vi "Auton Lift Dictation.vi"(1 "Level":dbl, 2 "First Iteration":bool) -> (0 "Lift Sequence Done":bool)   [LabVIEW 2014]
uses:
  Begin/Global Variables.vi
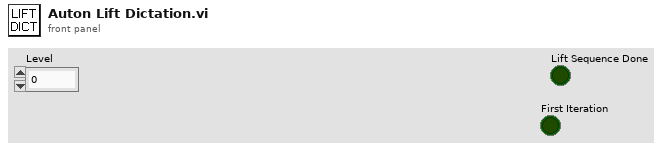
[diagram p1: front panel]
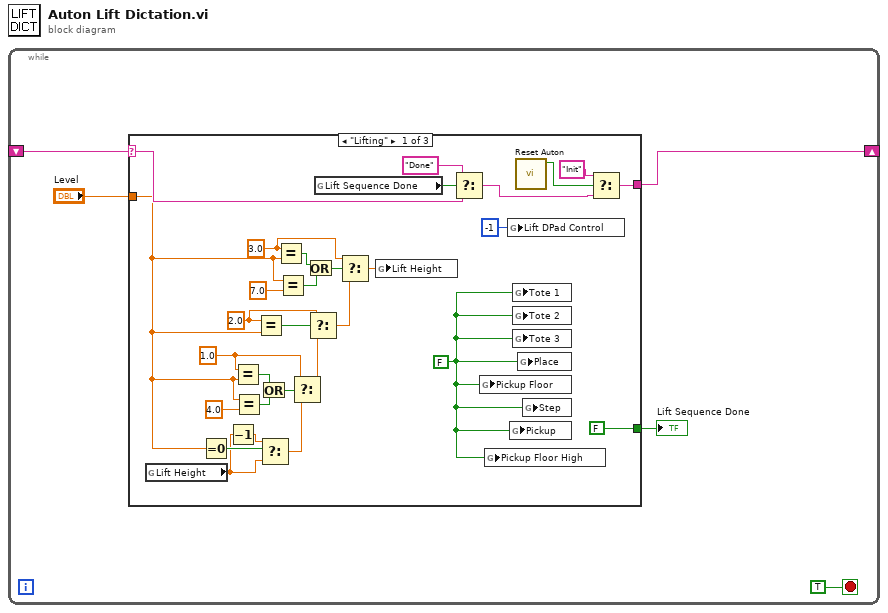
[diagram p0: block diagram]
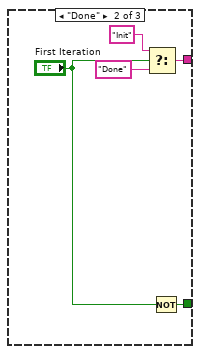
[diagram p2: hidden frame]
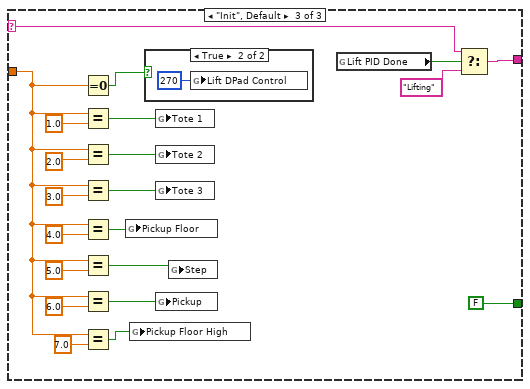
[diagram p3: hidden frame]
diagram:
  n1 = while {
    shift-right: [w1] -> _
    shift-left: _ -> [w2]
    stop <- TRUE stop-if-true
    n2 = case shown="\"Lifting\"" w2 {
      selector: w2 -> [w34 _ w46]
      tunnel: "Level" -> [w15 _ w43]
      tunnel: [w9 w39 w49] -> w1
      tunnel: [FALSE ("Lift Sequence Done") w37 FALSE ("Lift Sequence Done")] -> w4
      frame "Lifting" {
        w11 = 3.0 ("x")
        w22 = 2.0 ("x")
        w25 = 1.0 ("x")
        w30 = FALSE ("Tote 0")
        n3 = global read "Global Variables.vi" "Lift Height"() -> (w26:dbl)
        n4 = Equal To 0?(x=w15) -> (x = 0?=w29:bool)
        n5 = Decrement(x=w26) -> (x-1=w27:dbl)
        n6 = Equal?(x=w25, y=w15) -> (x = y?=w18:bool)
        n7 = Equal?(x=w15, y=4.0) -> (x = y?=w19:bool)
        n8 = Equal?(x=w22, y=w15) -> (x = y?=w23:bool)
        n9 = Or(x=w18, y=w19) -> (x .or. y?=w17:bool)
        n10 = Select(t=w27, s=w29, f=w26) -> (s? t:f=w28:dbl)
        n11 = Equal?(x=w11, y=w15) -> (x = y?=w13:bool)
        n12 = Equal?(x=w15, y=7.0 ("x")) -> (x = y?=w14:bool)
        n13 = Select(t=w25, s=w17, f=w28) -> (s? t:f=w24:dbl)
        n14 = Or(x=w13, y=w14) -> (x .or. y?=w12:bool)
        n15 = Select(t=w22, s=w23, f=w24) -> (s? t:f=w21:dbl)
        n16 = global read "Global Variables.vi" "Lift Sequence Done"() -> (w35:bool)
        n17 = Select(t=w11, s=w12, f=w21) -> (s? t:f=w10:dbl)
        n18 = global write "Global Variables.vi" "Lift Height"(w10) -> ()
        n19 = Select(t="Done", s=w35, f=w34) -> (s? t:f=w8:string)
        n20 = global write "Global Variables.vi" "Pickup Floor"(w30) -> ()
        n21 = global write "Global Variables.vi" "Pickup Floor High"(w30) -> ()
        n22 = global write "Global Variables.vi" "Lift DPad Control"(i16 -1 ("Lift DPad Control")) -> ()
        n23 = global write "Global Variables.vi" "Pickup"(w30) -> ()
        n24 = global write "Global Variables.vi" "Tote 1"(w30) -> ()
        n25 = global write "Global Variables.vi" "Tote 2"(w30) -> ()
        n26 = global write "Global Variables.vi" "Tote 3"(w30) -> ()
        n27 = call "Reset Auton.vi"() -> ("Reset Auton"=w7:bool)  [unwired: 11 in]
        n28 = global write "Global Variables.vi" "Place"(w30) -> ()
        n29 = global write "Global Variables.vi" "Step"(w30) -> ()
        n30 = Select(t="Init", s=w7, f=w8) -> (s? t:f=w9:string)
      }
      frame "Done" {
        n31 = Select(t="Init" ("f"), s="First Iteration", f="Done") -> (s? t:f=w39:string)
        n32 = Not(x="First Iteration") -> (.not. x?=w37:bool)
      }
      frame "Init", Default {
        n33 = Equal To 0?(x=w43) -> (x = 0?=w44:bool)
        n34 = Equal?(x=w43, y=1.0 ("x")) -> (x = y?=w60:bool)
        n35 = Equal?(x=w43, y=2.0 ("x")) -> (x = y?=w59:bool)
        n36 = Equal?(x=w43, y=3.0 ("x")) -> (x = y?=w61:bool)
        n37 = Equal?(x=w43, y=4.0) -> (x = y?=w58:bool)
        n38 = Equal?(x=w43, y=5.0) -> (x = y?=w55:bool)
        n39 = Equal?(x=w43, y=6.0) -> (x = y?=w54:bool)
        n40 = Equal?(x=w43, y=7.0) -> (x = y?=w41:bool)
        n41 = global write "Global Variables.vi" "Pickup Floor"(w58) -> ()
        n42 = global write "Global Variables.vi" "Pickup Floor High"(w41) -> ()
        n43 = case shown="True" w44 {
          frame False {
          }
          frame True {
            n44 = global write "Global Variables.vi" "Lift DPad Control"(i16 270 ("Lift DPad Control")) -> ()
          }
        }
        n45 = global write "Global Variables.vi" "Tote 1"(w60) -> ()
        n46 = global write "Global Variables.vi" "Tote 2"(w59) -> ()
        n47 = global write "Global Variables.vi" "Tote 3"(w61) -> ()
        n48 = global write "Global Variables.vi" "Pickup"(w54) -> ()
        n49 = global write "Global Variables.vi" "Step"(w55) -> ()
        n50 = global read "Global Variables.vi" "Lift PID Done"() -> (w48:bool)
        n51 = Select(t=w46, s=w48, f="Lifting") -> (s? t:f=w49:string)
      }
    }
    "Lift Sequence Done" <- w4
  }
